vi "Initialize.vi"(8 "error in (no error)":errorcluster, 9 "VISA Com Port":refnum<visa-resource-name>, 10 "Serial Device Brand":T1, 11 "Cypress in":refnum<class "Cypress.lvclass">) -> (0 "error out":errorcluster, 3 "Cypress out":refnum<class "Cypress.lvclass">)   [LabVIEW 2020, in "Cypress.lvclass"]
doc: "Método heredado del padre con un override"
uses:
  Cypress.lvclass
  Controles/Brand combobox.ctl
  <vilib>/Instr/_visa.llb/VISA Configure Serial Port (Instr).vi
  Abstract/Serial device/Serial device.lvclass
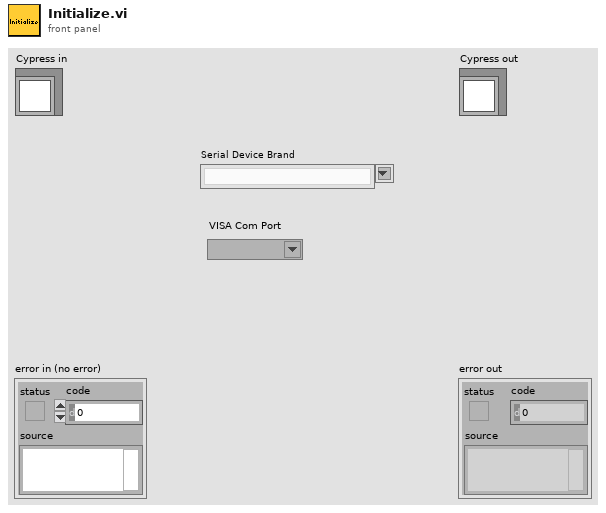
[diagram p1: front panel]
types:
  T1 = typedef "Serial device.lvclass/Brand combobox.ctl" = string
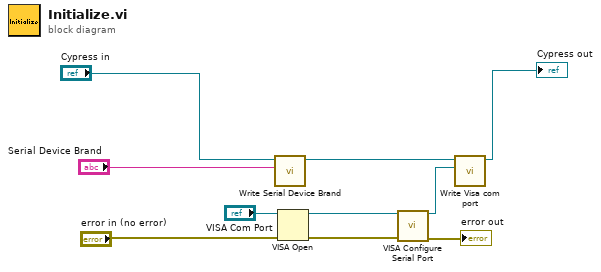
[diagram p0: block diagram]
diagram:
  n1 = call-dynamic "Write Serial Device Brand.vi"("Serial Device Brand"="Serial Device Brand", "Serial device in"="Cypress in") -> ("Serial device out"=w2:refnum<class "Cypress.lvclass">)  [unwired: 8 in, 1 out]
  n2 = VISA Open(error in (no error)="error in (no error)", VISA resource name="VISA Com Port") -> (VISA resource name=w4:refnum<visa-resource-name>, error out=w7:errorcluster)  [unwired: 3 in]
  n3 = call-poly "VISA Configure Serial Port"("VISA resource name"=w4, "error in (no error)"=w7) -> ("VISA resource name out"=w3:refnum<visa-resource-name>, "error out"=→"error out":errorcluster)  [unwired: 12 in]
  n4 = call-dynamic "Write Visa com port.vi"("Visa com port"=w3, "Serial device in"=w2) -> ("Serial device out"=→"Cypress out":refnum<class "Cypress.lvclass">)  [unwired: 8 in, 1 out]
